vi "AutonomousFeedback.vi"(8 "error in":errorcluster) -> ()   [LabVIEW 2015]
uses:
  <vilib>/Rock Robotics/Network Tables/NT Read Boolean.vi
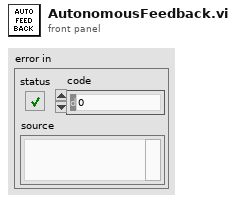
[diagram p1: front panel]
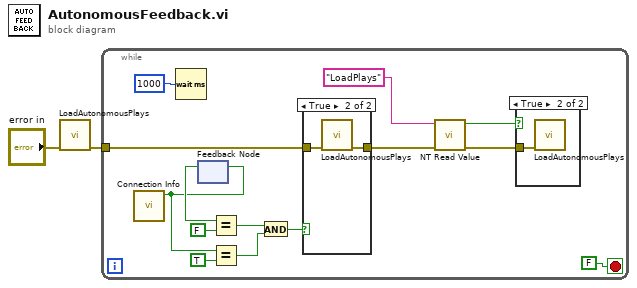
[diagram p0: block diagram]
diagram:
  n1 = call "LoadAutonomousPlays.vi"("error in"="error in") -> ("error out"=w1:errorcluster)  [unwired: 10 in]
  n2 = while {
    tunnel: w1 -> [w4]
    stop <- FALSE stop-if-true
    n3 = call <vilib>:"Connection Info.vi"() -> ("Connected"=w8:bool)  [unwired: 10 in, 1 out]
    n4 = Wait (ms)(milliseconds to wait=u32 1000) -> ()  [unwired: 1 out]
    n5 = feedback-in #1(w8) -> ()
    n6 = feedback #1() -> (w11:bool)  [unwired: 1 in]
    n7 = Equal?(x=w11, y=FALSE) -> (x = y?=w7:bool)
    n8 = Equal?(x=w8, y=TRUE) -> (x = y?=w6:bool)
    n9 = And(x=w7, y=w6) -> (x .and. y?=w5:bool)
    n10 = case shown="True" w5 {
      tunnel: w4 -> [w17 w19]
      tunnel: [w17 w18] -> w3
      frame False {
      }
      frame True {
        n11 = call "LoadAutonomousPlays.vi"("error in"=w19) -> ("error out"=w18:errorcluster)  [unwired: 10 in]
      }
    }
    n12 = call-poly <vilib>:"NT Read Value.vi"("error in"=w3, "Name"="LoadPlays") -> ("error out"=w12:errorcluster, "Boolean"=w14:bool)  [unwired: 8 in]
    n13 = case shown="True" w14 {
      tunnel: w12 -> [_ w20]
      frame False {
      }
      frame True {
        n14 = call "LoadAutonomousPlays.vi"("error in"=w20) -> ()  [unwired: 10 in, 1 out]
      }
    }
  }
